vi "Waveform Attribute, Get Timestamp.vi"(6 "error in":errorcluster, 9 "waveform":waveform(dbl)={"t0"=timestamp(3473168073.631 s since 1904-01-01), "dt"=1e-08, "Y"=[], "attributes"=variant("Average Size"=variant(dbl 15.0), "Frequency (Hz)"=variant(dbl 1998.0121510714948), "MD5[0]"=variant(dbl 3432209604.0), "MD5[1]"=variant(dbl 1216260660.0), "MD5[2]"=variant(dbl 1007192998.0), "MD5[3]"=variant(dbl 1264973305.0), "NSamp"=variant(dbl 400000.0), "Process Timestamp"=variant(timestamp timestamp(3473980972.5625 s since 1904-01-01)), "Recvy Amp (V)"=variant(dbl 2.6380060214865355), "Recvy Amp (mA)"=variant(dbl 5.276012042973071), "Recvy Frequency (Hz)"=variant(dbl 1998.1569402889318), "Recvy Pulse Width (us)"=variant(dbl 12.43212812423706), "Recvy Trigger (s)"=variant(dbl 0.00044001), "Resistance (ohms)"=variant(dbl 500.0), "Samp Freq (MHz)"=variant(dbl 100.0), "Stim Amp (V)"=variant(dbl -2.3028964175483475), "Stim Amp (mA)"=variant(dbl -4.605792835096695), "Stim Frequency (Hz)"=variant(dbl 1997.8673618540577), "Stim Pulse Width (us)"=variant(dbl 12.074634451866151), "Stim Trigger (s)"=variant(dbl 0.00041214), "dt (us)"=variant(dbl 0.01))}) -> (0 "error out":errorcluster, 1 "Process Timestamp":dbl[unit]=nan format="%.3f", 3 "waveform dup":waveform(dbl)={"t0"=timestamp(0 s since 1904-01-01), "dt"=nan, "Y"=[]}, 4 "Date and Time":timestamp=timestamp(-9593226000 s since 1904-01-01) format="%<%.1X  %x>T ")   [LabVIEW 2010]
doc: "The timestamp is the current time in seconds. LabVIEW calculates this timestamp using the number of seconds elapsed since 12:00 a.m., Friday, January 1, 1904, Universal Time [01-01-1904 00:00:00]."
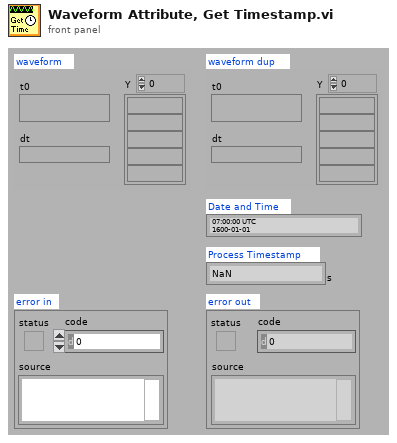
[diagram p1: front panel]
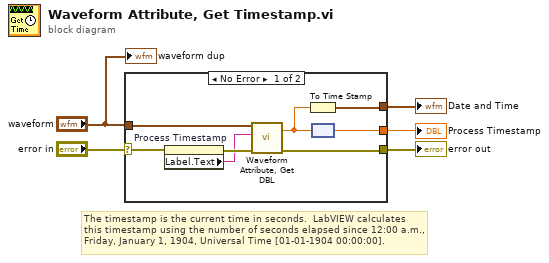
[diagram p0: block diagram]
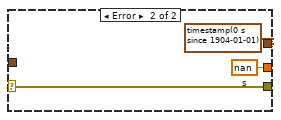
[diagram p2: hidden frame]
diagram:
  # "The timestamp is the current time in seconds.  LabVIEW calculates this timestamp using the number of seconds elapsed since 12:00 a.m., Friday, January 1, 1904, Universal Time [01-01-1904 00:00:00]."
  n1 = case shown="No Error" "error in" {
    selector: "error in" -> [w11 w16]
    tunnel: [w7 w16] -> w5
    tunnel: "waveform" -> [w8 _]
    tunnel: [w13 w15] -> w2
    tunnel: [w12 timestamp(0 s since 1904-01-01) ("Process Timestamp 2")] -> w1
    frame No Error {
      n2 = property on="Process Timestamp" class="DigNum (strict)"(error in=w11) -> (error out=w10:errorcluster, "Label.Text"=w9:string)  [unwired: 1 in, 1 out]
      n3 = call "Waveform Attribute, Get DBL.vi"("error in"=w10, "label"=w9, "waveform"=w8) -> ("error out"=w7:errorcluster, "value"=w6:dbl)  [unwired: 3 in, 2 out]
      n4 = To Time Stamp(1:w6) -> (0:w12:timestamp)
      n5 = node(w6) -> (w13:dbl[unit])
    }
    frame Error {
      w15 = dbl[unit] nan  # s
    }
  }
  "error out" <- w5
  "Date and Time" <- w1
  "Process Timestamp" <- w2
  "waveform dup" <- "waveform"
